vi "Connect.vi"(8 "error in (no error)":errorcluster, 9 "timeout":i32=-1, 11 "TCP Stream Listener in":refnum<class "TCP Stream Listener.lvclass">) -> (0 "error out":errorcluster, 3 "TCP Stream Listener out":refnum<class "TCP Stream Listener.lvclass">)   [LabVIEW 2020, in "TCP Stream Listener.lvclass"]
doc: "This method waits for a remote connection from a TCP/IP Stream Initiator."
uses:
  TCP Stream Listener.lvclass
  TCP Stream/TCP Stream.lvclass
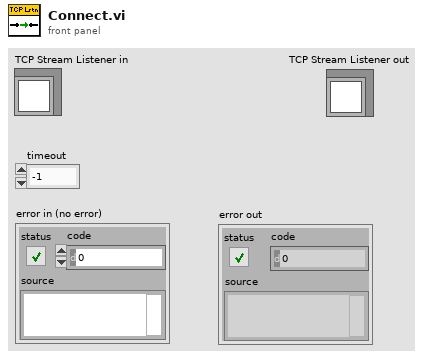
[diagram p1: front panel]
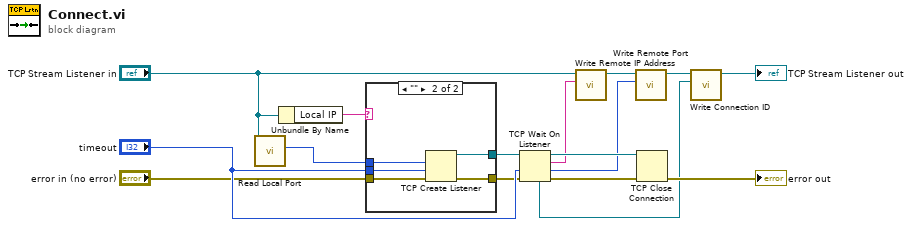
[diagram p0: block diagram]
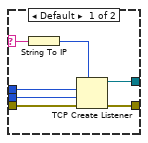
[diagram p2: hidden frame]
diagram:
  n1 = call "Read Local Port.vi"("TCP Stream in"="TCP Stream Listener in") -> ("local port"=w6:u16)  [unwired: 10 in]
  n2 = Unbundle By Name("TCP Stream Listener in") -> ("Local IP"=w1:string)
  n3 = case shown="\"\"" w1 {
    selector: w1 -> [w18 _]
    tunnel: "timeout" -> [w22 w28]
    tunnel: "error in (no error)" -> [w23 w27]
    tunnel: [w19 w26] -> w11
    tunnel: [w20 w25] -> w10
    tunnel: w6 -> [w21 w24]
    frame Default {
      n4 = String To IP(1:w18) -> (0:w17:u32)
      n5 = TCP Create Listener(7:w17, 8:w23, 9:w22, 10:w21) -> (0:w19:errorcluster, 3:w20:refnum<k5>)  [unwired: 1 in, 1 out]
    }
    frame "" {
      n6 = TCP Create Listener(8:w27, 9:w28, 10:w24) -> (0:w26:errorcluster, 3:w25:refnum<k5>)  [unwired: 2 in, 1 out]
    }
  }
  n7 = TCP Wait On Listener(8:w11, 9:"timeout", 11:w10) -> (0:w9:errorcluster, 1:w2:u16, 2:w3:string, 3:w8:refnum<k5>, 4:w7:refnum<k5>)  [unwired: 1 in]
  n8 = call "Write Remote IP Address.vi"("Remote IP"=w3, "TCP Stream in"="TCP Stream Listener in") -> ("TCP Stream out"=w5:refnum<class "TCP Stream Listener.lvclass">)  [unwired: 9 in]
  n9 = call "Write Remote Port.vi"("remote port"=w2, "TCP Stream in"=w5) -> ("TCP Stream out"=w4:refnum<class "TCP Stream Listener.lvclass">)  [unwired: 9 in]
  n10 = TCP Close Connection(connection ID=w8, error in (no error)=w9) -> (error out=→"error out":errorcluster)  [unwired: 1 in, 1 out]
  n11 = call "Write Connection ID.vi"("connection ID"=w7, "TCP Stream in"=w4) -> ("TCP Stream out"=→"TCP Stream Listener out":refnum<class "TCP Stream Listener.lvclass">)  [unwired: 9 in]
